vi "Test Customer with Phone Make Call Broadcasts Status.vi"(8 "error in (no error)":errorcluster, 11 "Customer With Phone Test In":refnum<class "Customer With Phone Test.lvclass">=refnum) -> (0 "error out":errorcluster, 3 "Customer With Phone Test Out":refnum<class "Customer With Phone Test.lvclass">)   [LabVIEW 2020, in "Customer With Phone Test.lvclass"]
uses:
  Customer With Phone Test.lvclass
  <vilib>/Astemes/Triarc Framework/Process/Process.lvclass
  Processes/People/Customers/Customer With Phone/Customer With Phone.lvclass
  C:/git/astemes-triarc-examples/source/Coffee Shop/Processes/People/Customers/Customer/Customer.lvclass
  C:/git/astemes-triarc-examples/source/Coffee Shop/Processes/People/Person/Person.lvclass
  C:/Program Files (x86)/National Instruments/LabVIEW 2020/vi.lib/Astemes/Triarc Framework/View/View.lvclass
  C:/Program Files (x86)/National Instruments/LabVIEW 2020/vi.lib/Astemes/Triarc Framework/Process/Process.lvclass
  C:/Program Files (x86)/National Instruments/LabVIEW 2020/vi.lib/Astemes/Triarc Framework/Base/Base.lvclass
  C:/Program Files (x86)/National Instruments/LabVIEW 2020/vi.lib/Astemes/Triarc Framework/Error Handler Interface/Error Handler Interface.lvclass
  C:/Program Files (x86)/National Instruments/LabVIEW 2020/vi.lib/Astemes/Triarc Framework/Logging/Logging.lvclass
  C:/git/astemes-triarc-examples/source/Coffee Shop/Processes/People/Process Job/Job Handler.lvclass
  C:/Program Files (x86)/National Instruments/LabVIEW 2020/vi.lib/Astemes/Triarc Framework/Async Handler/Async Handler.lvclass
  C:/git/astemes-triarc-examples/source/Coffee Shop/Processes/People/Customers/Customer With Phone/Customer With Phone.lvclass
  C:/Program Files (x86)/National Instruments/LabVIEW 2020/vi.lib/Astemes/Triarc Framework/Helper Loop/Helper Loop.lvclass
  84041711-a98c-4458-8a7e-b29b434b9d89.vi
  <vilib>/Astemes/Triarc Framework/Support/Broadcast Event Dequeuers.lvlib
  <vilib>/Astemes/LUnit/Test Case.lvclass
  C:/Program Files (x86)/National Instruments/LabVIEW 2020/vi.lib/Astemes/LUnit/Test Case.lvclass
  C:/Program Files (x86)/National Instruments/LabVIEW 2020/vi.lib/Astemes/LUnit/LUnit Runnable.lvclass
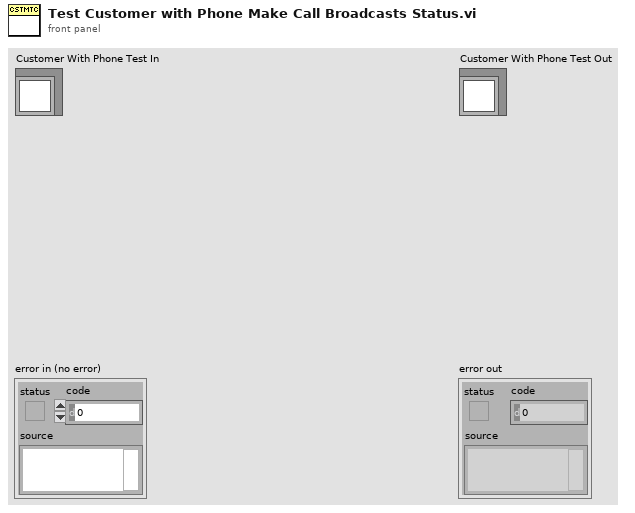
[diagram p1: front panel]
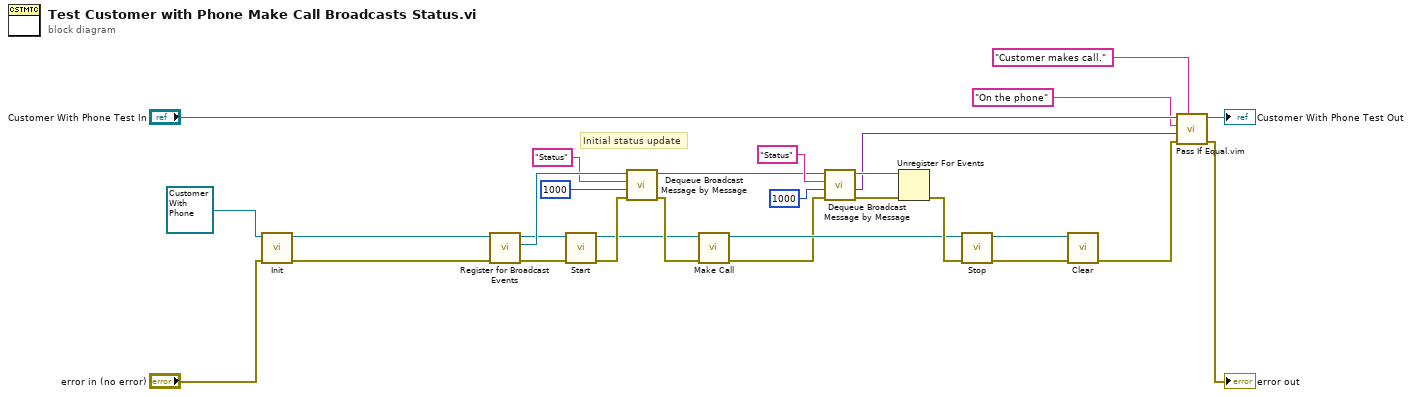
[diagram p0: block diagram]
diagram:
  # "Initial status update"
  n1 = call-dynamic "Init.vi"("error in (no error)"="error in (no error)", "View In"=refnum<class "Customer With Phone.lvclass"> refnum ("Customer With Phone.lvclass")) -> ("error out"=w29:errorcluster, "View Out"=w24:refnum<class "Customer With Phone.lvclass">)  [unwired: 8 in]
  n2 = call <vilib>:"Register for Broadcast Events.vi"("error in (no error)"=w29, "Process In"=w24) -> ("error out"=w6:errorcluster, "Event Registration Refnum Out"=w9:refnum<event-registration>, "Process Out"=w3:refnum<class "Customer With Phone.lvclass">)  [unwired: 7 in]
  n3 = call <vilib>:"Start.vi"("error in (no error)"=w6, "Process In"=w3) -> ("error out"=w4:errorcluster, "Process Out"=w2:refnum<class "Customer With Phone.lvclass">)  [unwired: 7 in, 1 out]
  n4 = call <vilib>:"Dequeue Broadcast Message by Message.vi"("error in (no error)"=w4, "Timeout (-1)"=1000, "Message"="Status", "Event Registration Refnum"=w9) -> ("error out"=w5:errorcluster, "Event Registration Refnum Out"=w8:refnum<event-registration>)  [unwired: 3 in, 3 out]
  n5 = call "Make Call.vi"("error in (no error)"=w5, "Customer With Phone In"=w2) -> ("error out"=w11:errorcluster, "Customer With Phone Out"=w27:refnum<class "Customer With Phone.lvclass">)  [unwired: 8 in]
  n6 = call <vilib>:"Dequeue Broadcast Message by Message.vi"("error in (no error)"=w11, "Timeout (-1)"=1000, "Message"="Status", "Event Registration Refnum"=w8) -> ("error out"=w10:errorcluster, "Message Data"=w14:variant, "Event Registration Refnum Out"=w15:refnum<event-registration>)  [unwired: 3 in, 2 out]
  n7 = Unregister For Events(event registration refnum=w15, error in=w10) -> (error out=w28:errorcluster)
  n8 = call <vilib>:"Stop.vi"("error in (no error)"=w28, "Process In"=w27) -> ("error out"=w26:errorcluster, "Process Out"=w25:refnum<class "Customer With Phone.lvclass">)  [unwired: 7 in, 1 out]
  n9 = call-dynamic "Clear.vi"("error in (no error)"=w26, "View In"=w25) -> ("error out"=w17:errorcluster)  [unwired: 9 in]
  n10 = call "Pass If Equal.vim"("Description"="Customer makes call.", "error in (no error)"=w17, "Actual"=w14, "Expected"="On the phone", "LUnit Test Case In"="Customer With Phone Test In") -> ("error out"=→"error out":errorcluster, "LUnit Test Case Out"=→"Customer With Phone Test Out":refnum<class "Test Case.lvclass">)  [unwired: 5 in]
